vi "DQMH Load Main VI Reference.vi"(8 "error in (no error)":errorcluster, 11 "VI in":refnum<vi>) -> (0 "error out":errorcluster, 2 "Execution:State":T1(ring), 3 "VI out":refnum<vi>)   [LabVIEW 2020, in "hse-dqmh.lvlib"]
doc: "Loads the VI reference to a Singleton DQMH module's main.vi. On Linux RT in Runtime Environment, the main.vi is loaded reentrant in order to circumevent a bug in LabVIEW.\n\nDetails: On Linux RT with Embedded UI enabled running a startup.exe, a VI server invoke method (Control Value.set) doesn't work. This is possibly related to / covered by CAR 514879 (see\nhttps://forums.ni.com/t5/Delacor-Toolkits-Discussions/Deploy-and-run-at-Startup-for-RT-systems/m-p/3620339/highlight/true#M256).\n\nIn order for this VI to work, you need to:\n1. set the DQMH module's main.vi execution setting to \"preallocated clone reentrant execution\"\n2. set the DQMH module's main.vi scope to \"community\"\n3. add the hse-dqmh.lvlib as a friend in the DQMH module's .lvlib Friends properties\n\n____\nHAMPEL SOFTWARE ENGINEERING v3.8.0 (2023-12-18 14:41)"
uses:
  hse-dqmh.lvlib
  hse-misc/hse-misc.lvlib
panel:
  # "Loads the VI reference to a Singleton DQMH module's main.vi. On Linux RT in Runtime Environment, the main.vi is loaded reentrant in order to circumevent a bug in LabVIEW.\n\nDetails: On Linux RT with Embedded UI enabled running a startup.exe, a VI server invoke method (Control Value.set) doesn't work. This is possibly related to / covered by CAR 514879 (see\nhttps://forums.ni.com/t5/Delacor-Toolkits-Discussions/Deploy-and-run-at-Startup-for-RT-systems/m-p/3620339/highlight/true#M256).\n\nIn order for this VI to work, you need to:\n1. set the DQMH module's main.vi execution setting to \"preallocated clone reentrant execution\"\n2. set the DQMH module's main.vi scope to \"community\"\n3. add the hse-dqmh.lvlib as a friend in the DQMH module's .lvlib Friends properties"
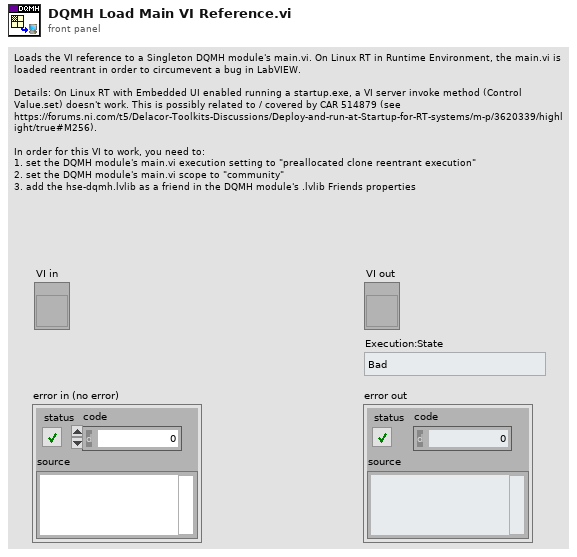
[diagram p1: front panel]
types:
  T1 = enum32{"Bad", "Idle", "Run top level", "Running"}
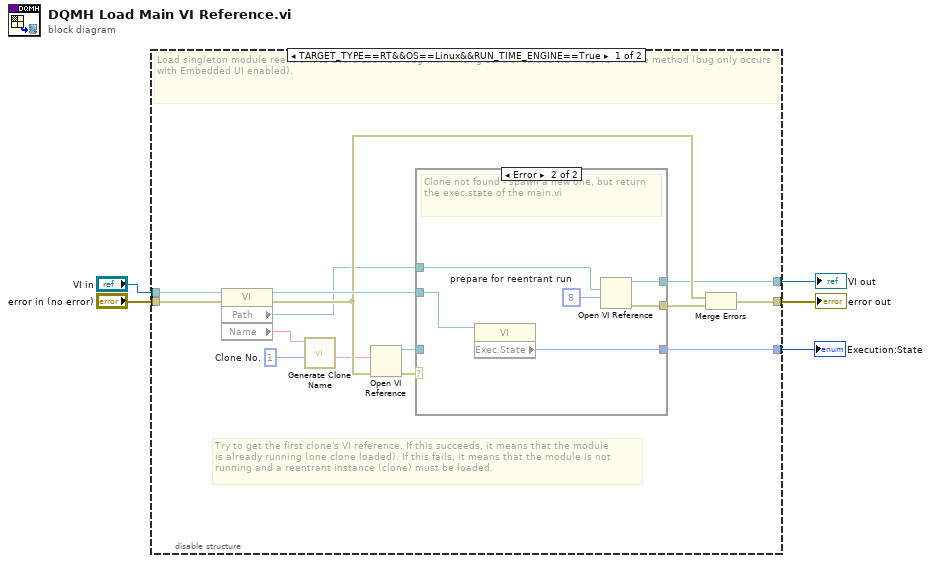
[diagram p0: block diagram]
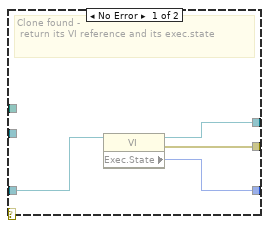
[diagram p2: hidden frame]
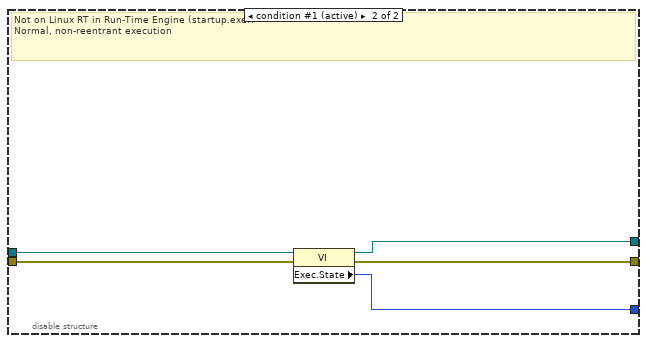
[diagram p3: hidden frame]
diagram:
  n1 = disable-structure shown="TARGET_TYPE==RT&&OS==Linux&&RUN_TIME_ENGINE==True" {
    disable-tunnel: "error in (no error)" -> [w9 w34]
    disable-tunnel: "VI in" -> [w8 w33]
    disable-tunnel: [w10 w31] -> w4
    disable-tunnel: [w11 w32] -> w2
    disable-tunnel: [w12 w30] -> w1
    frame condition #0 {
      w14 = 1  # Clone No.
      # "Try to get the first clone's VI reference. If this succeeds, it means that the module\nis already running (one clone loaded). If this fails, it means that the module is not\nrunning and a reentrant instance (clone) must be loaded."
      # "Load singleton module reentrant to avoid LabVIEW bug with writing control values via VI server invoke method (bug only occurs with Embedded UI enabled)."
      n2 = property class="VI"(reference=w8, error in=w9) -> (reference out=w19:refnum<vi>, error out=w17:errorcluster, "Path"=w7:path, "Name"=w13:string)
      n3 = call "Generate Clone Name.vi"("Clone number (1)"=w14, "Fully qualified VI name"=w13) -> ("Fully qualified clone name"=w6:string)  [unwired: 7 in, 2 out]
      n4 = Open VI Reference(vi path=w6, error in (no error)=w17) -> (vi reference=w16:refnum<vi>, error out=w15:errorcluster)  [unwired: 4 in]
      n5 = case shown="Error" w15 {
        tunnel: w7 -> [_ w29]
        tunnel: w16 -> [w23 _]
        tunnel: [w22 w27] -> w11
        tunnel: [w21 w24] -> w12
        tunnel: [w20 w26] -> w18
        tunnel: w19 -> [_ w25]
        frame No Error {
          # "Clone found -\n return its VI reference and its exec.state"
          n6 = property class="VI"(reference=w23) -> (reference out=w22:refnum<vi>, error out=w20:errorcluster, "Exec.State"=w21:T1)  [unwired: 1 in]
        }
        frame Error {
          w28 = 8  # prepare for reentrant run
          # "Clone not found - spawn a new one, but return the exec.state of the main.vi"
          n7 = property class="VI"(reference=w25) -> ("Exec.State"=w24:T1)  [unwired: 1 in, 2 out]
          n8 = Open VI Reference(vi path=w29, options=w28) -> (vi reference=w27:refnum<vi>, error out=w26:errorcluster)  [unwired: 4 in]
        }
      }
      n9 = Merge Errors(w17, w18) -> (w10:errorcluster)
    }
    frame condition #1 (active) {
      # "Not on Linux RT in Run-Time Engine (startup.exe): \nNormal, non-reentrant execution"
      n10 = property class="VI"(reference=w33, error in=w34) -> (reference out=w32:refnum<vi>, error out=w31:errorcluster, "Exec.State"=w30:T1)
    }
  }
  "error out" <- w4
  "VI out" <- w2
  "Execution:State" <- w1
